vi "PLC.Dial750, Look Up Symbols.vi"(8 "error in (no error)":errorcluster, 10 "VarNames In":T2={"SN"="g.SN", "Nest"="g.Nest", "Ready"="g.Ready", "Start"="g.Start", "Pass"="g.Pass", "Done"="g.Done", "Running"="GVL.gDone"}, 11 "Symbols In":T1[](array[typedef]) {"Index Offset" format="%.0x"; "Index Group" format="%.0x"}) -> (0 "error out":errorcluster, 3 "Var Info":T1[](array[typedef]) {"Index Offset" format="%.0x"; "Index Group" format="%.0x"})   [LabVIEW 2018]
uses:
  Controls/PLC750.Variable Names.ctl
  <instrlib>/_Ackermann Automation/TwinCAT ADS Library/TcAdsLV_Common/TypeDefs/ClusterAdsSymbolEntry.ctl
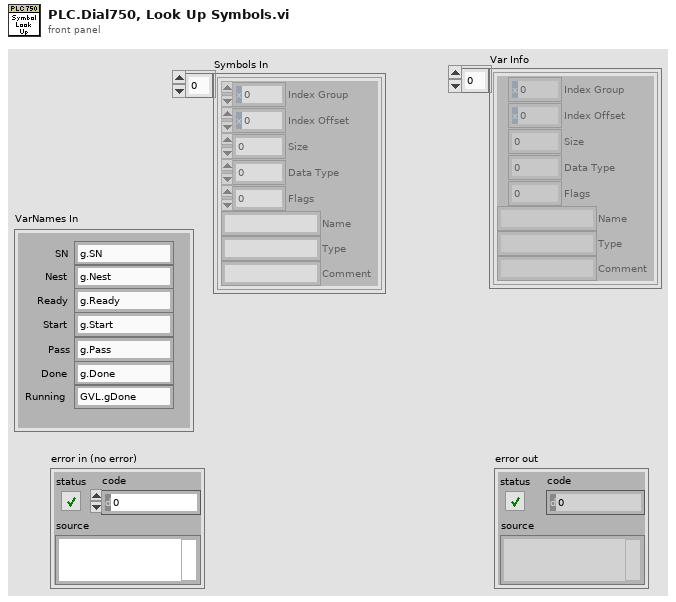
[diagram p1: front panel]
types:
  T1 = typedef "TcAdsLV_Common_3.lvlib/ClusterAdsSymbolEntry.ctl" = cluster{"Index Group":u32, "Index Offset":u32, "Size":u32, "Data Type":u32, "Flags":u32, "Name":string, "Type":string, "Comment":string}
  T2 = typedef "PLC750.Variable Names.ctl" = cluster{"SN":string, "Nest":string, "Ready":string, "Start":string, "Pass":string, "Done":string, "Running":string}
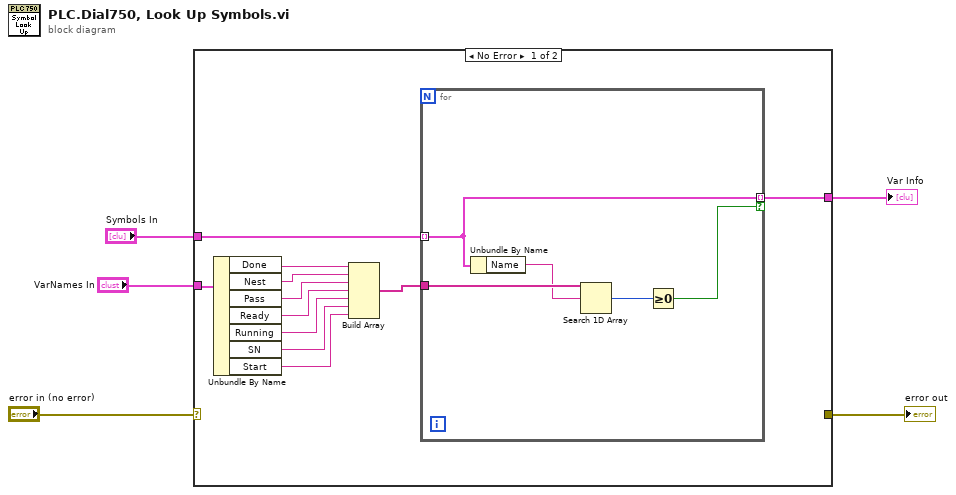
[diagram p0: block diagram]
diagram:
  n1 = case shown="No Error" "error in (no error)" {
    selector: "error in (no error)" -> [_ w22]
    tunnel: [_ w22] -> w4
    tunnel: "VarNames In" -> [w14 _]
    tunnel: [w16 _] -> w1
    tunnel: "Symbols In" -> [w15 _]
    frame No Error {
      n2 = Unbundle By Name(w14) -> ("Done"=w13:string, "Nest"=w12:string, "Pass"=w11:string, "Ready"=w10:string, "Running"=w9:string, "SN"=w8:string, "Start"=w7:string)
      n3 = Build Array(w13, w12, w11, w10, w9, w8, w7) -> (w6:string[])
      n4 = for {
        tunnel: w6 -> [w21]
        tunnel: [w20] -> w16 mode=indexing if=w19
        tunnel: w15 -> [w20] mode=indexing
        n5 = Unbundle By Name(w20) -> ("Name"=w18:string)
        n6 = Search 1D Array(1D array=w21, element=w18) -> (index of element=w17:i32)  [unwired: 1 in]
        n7 = Greater Or Equal To 0?(x=w17) -> (x >= 0?=w19:bool)
      }
    }
    frame Error {
    }
  }
  "error out" <- w4
  "Var Info" <- w1
